vi "Combine Key with Modifiers.vi"(1 "Modifiers":T1[](array[typedef]), 2 "Key":string) -> (0 "Combined":string)   [LabVIEW 2021, in "Seq Edit Quick Drop.lvlib"]
uses:
  Seq Edit Quick Drop.lvlib
  Modifiers.ctl
  <vilib>/Utility/error.llb/whitespace.ctl
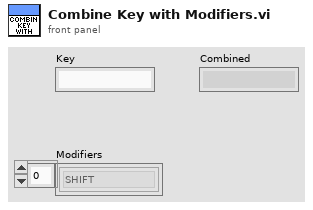
[diagram p1: front panel]
types:
  T1 = typedef "Seq Edit Quick Drop.lvlib/Modifiers.ctl" = enum16{"SHIFT", "CTRL", "ALT"}
  T2 = typedef "whitespace.ctl" = u16
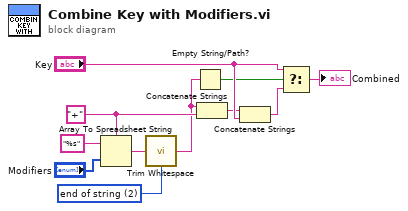
[diagram p0: block diagram]
diagram:
  w1 = T2 2 items=["both", "start of string", "end of string"] ("location (both)")
  w5 = "+" ("delimiter (Tab)")
  n1 = Array To Spreadsheet String(delimiter (Tab)=w5, array="Modifiers", 3:"%s" ("format string")) -> (spreadsheet string=w6:string)
  n2 = call <vilib>:"Trim Whitespace.vi"("string"=w6, "location (both)"=w1) -> ("trimmed string"=w2:string)
  n3 = Empty String/Path?(string/path=w2) -> (empty?=w7:bool)
  n4 = Concatenate Strings(w2, w5) -> (w8:string)
  n5 = Concatenate Strings(w8, "Key") -> (w10:string)
  n6 = Select(t="Key", s=w7, f=w10) -> (s? t:f=→"Combined":string)
